vi "SmartSEM Remote API FIB mag.vi"(8 "error in":errorcluster, 10 "FIB FOV (um)":sgl=500.0 format="%.3g", 11 "Api":refnum<k7>(container)) -> (0 "error out":errorcluster, 3 "Api out":refnum<k7>)   [LabVIEW 2018]
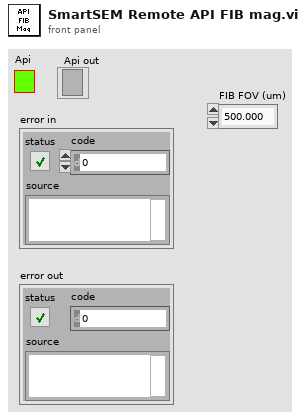
[diagram p1: front panel]
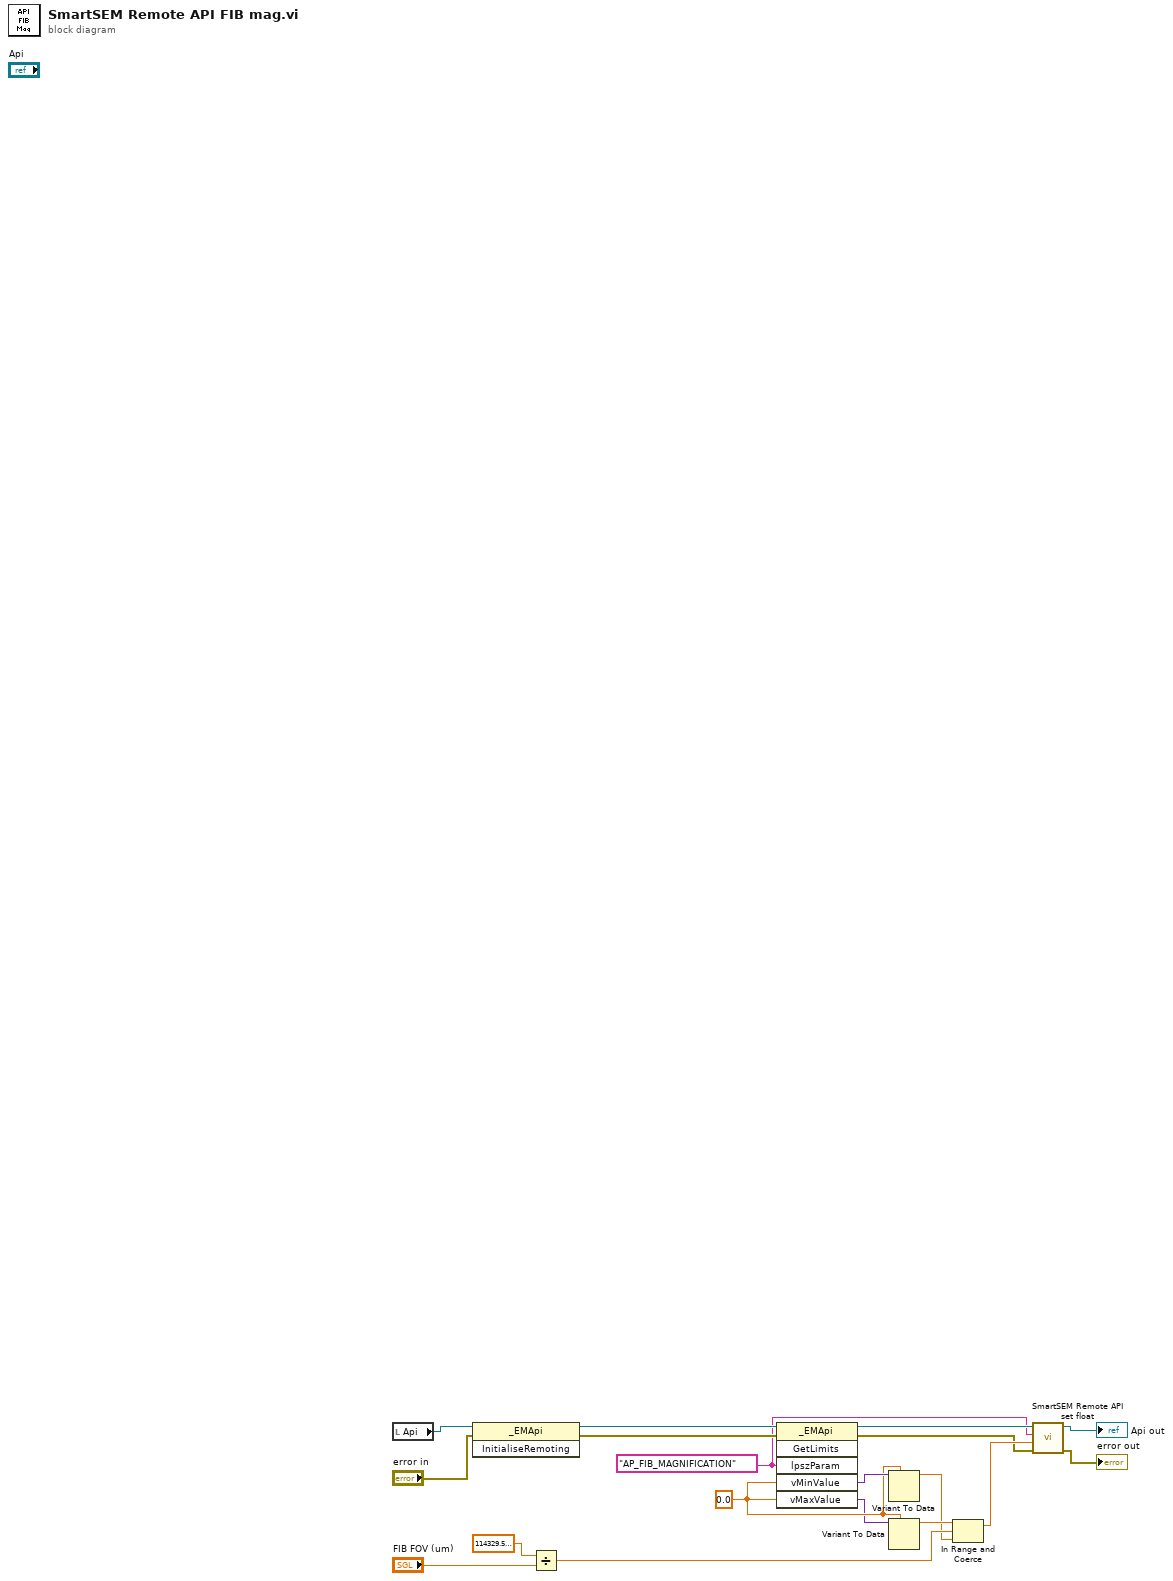
[diagram p0: block diagram]
diagram:
  w13 = sgl 0.0
  w5 = "AP_FIB_MAGNIFICATION" ("lpszParam")
  n1 = local read "Api"() -> (w18:refnum<k7>)
  n2 = invoke class="_EMApi" method="InitialiseRemoting"(reference=w18, error in="error in") -> (reference out=w16:refnum<k7>, error out=w15:errorcluster)  [unwired: 1 in, 1 out]
  n3 = Divide(x=sgl 114329.59, y="FIB FOV (um)") -> (x/y=w10:sgl)
  n4 = invoke class="_EMApi" method="GetLimits"(reference=w16, error in=w15, "lpszParam"=w5, "vMinValue"=w13, "vMaxValue"=w13) -> (reference out=w6:refnum<k7>, error out=w3:errorcluster, "vMinValue"=w14:variant, "vMaxValue"=w7:variant)  [unwired: 1 in, 2 out]
  n5 = Variant To Data(type=w13, Variant=w14) -> (data=w8:sgl)  [unwired: 1 in, 1 out]
  n6 = Variant To Data(type=w13, Variant=w7) -> (data=w9:sgl)  [unwired: 1 in, 1 out]
  n7 = In Range and Coerce(upper limit=w9, x=w10, lower limit=w8) -> (coerced(x)=w4:sgl)  [unwired: 1 out]
  n8 = call "SmartSEM Remote API set float.vi"("error in"=w3, "vValue"=w4, "lpszParam"=w5, "Api"=w6) -> ("error out"=→"error out":errorcluster, "Api out"=→"Api out":refnum<k7>)  [unwired: 6 in]
